vi "Diagnostic Global.vi"() -> ()   [LabVIEW 2013]
panel:
  in  "Diag_Global":fxp<+/-,28,17>[](array[numeric])=[0.0, 0.0, 0.0, 0.0, 0.0, 0.0]
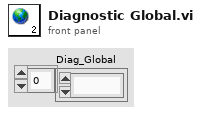
[diagram p1: front panel]
diagram:
